vi "sht41-csv-to-data.vi"(10 "sensor-name":string, 11 "sensor-csv-input":string) -> (1 "SHT41: Humidity (%)":dbl format="%.2f", 2 "SHT41: Temp (degC)":dbl format="%.2f", 3 "SHT41: data output":T1 {"Humidity (%)" format="%.2f"; "Temp (degC)" format="%.2f"})   [LabVIEW 2021]
uses:
  SHT41.ctl
  <vilib>/regexp/Match Regular Expression.xnode
panel:
  out "SHT41: Humidity":string
  out "SHT41: Temperature":string
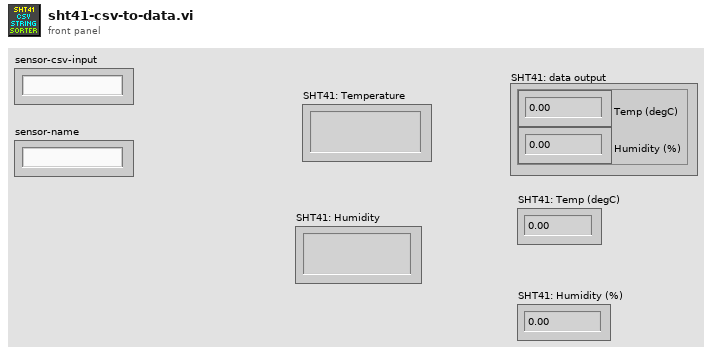
[diagram p1: front panel]
types:
  T1 = typedef "SHT41.ctl" = cluster{"Temp (degC)":dbl, "Humidity (%)":dbl}
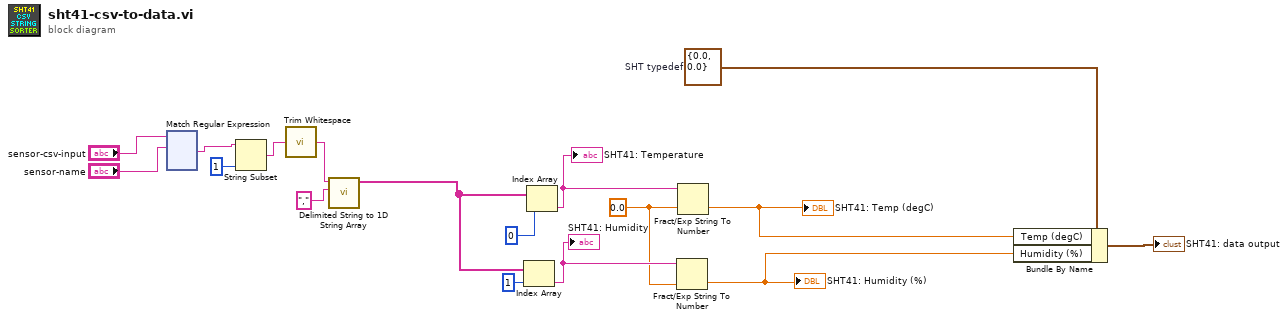
[diagram p0: block diagram]
diagram:
  w13 = T1 {"Temp (degC)"=0.0, "Humidity (%)"=0.0}  # SHT typedef
  w14 = 0.0
  n1 = xnode "Match Regular Expression"("input string"="sensor-csv-input", "regular expression"="sensor-name") -> ("after match"=w2:string)  [unwired: 4 in, 4 out]
  n2 = String Subset(string=w2, offset (0)=1) -> (substring=w1:string)  [unwired: 1 in]
  n3 = call <vilib>:"Trim Whitespace.vi"("string"=w1) -> ("trimmed string"=w9:string)  [unwired: 1 in]
  n4 = call <vilib>:"Delimited String to 1D String Array.vi"("delimiter"=",", "delimited string"=w9) -> ("string array"=w5:string[])  [unwired: 9 in]
  n5 = Index Array(array=w5, index=1) -> (element=w15:string)
  "SHT41: Humidity" <- w15
  n6 = Index Array "Index Array"(array=w5, index=0) -> (element=w16:string)
  "SHT41: Temperature" <- w16
  n7 = Fract/Exp String To Number(string=w15, default (0 dbl)=w14) -> (number=w11:dbl)  [unwired: 2 in, 1 out]
  "SHT41: Humidity (%)" <- w11
  n8 = Fract/Exp String To Number(string=w16, default (0 dbl)=w14) -> (number=w12:dbl)  [unwired: 2 in, 1 out]
  "SHT41: Temp (degC)" <- w12
  n9 = Bundle By Name(cluster=w13, "Temp (degC)"=w12, "Humidity (%)"=w11) -> (→"SHT41: data output":T1)
